vi "CT_DelayPMT_TL_trig.vi"(1 "TL Index":i32=5, 2 "Size of Trig Waveform":dbl=4000.0, 3 "PMT Trig Index":i32=2, 4 "Very Fast Timing In":dbl[](array[slide])=[1100.0, 3200.0, 3254.0, 3290.0, 3100.0, 3080.0, 0.0, 3100.0] min=0.0 max=4000.0 step=2.0 scale=0.0..4000.0 scale format="%#_3f") -> (0 "Very Fast Timing Out":dbl[](array[slide])=[1100.0, 3200.0, 3254.0, 3290.0, 3100.0, 3080.0, 0.0, 3100.0] min=0.0 max=4000.0 step=2.0 scale=0.0..4000.0 scale format="%#_3f")   [LabVIEW 2009]
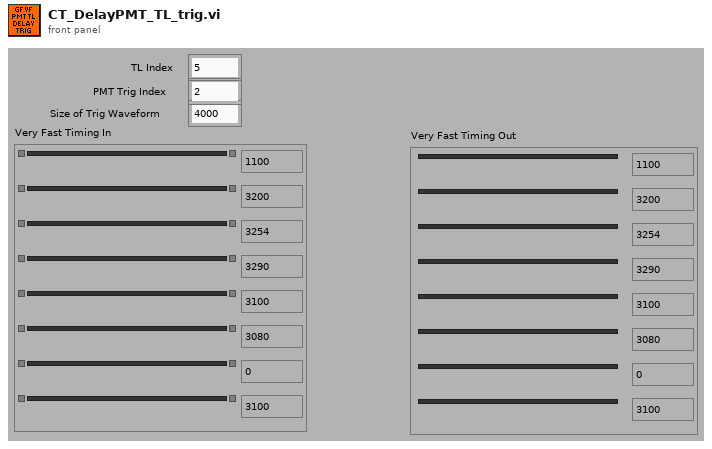
[diagram p1: front panel]
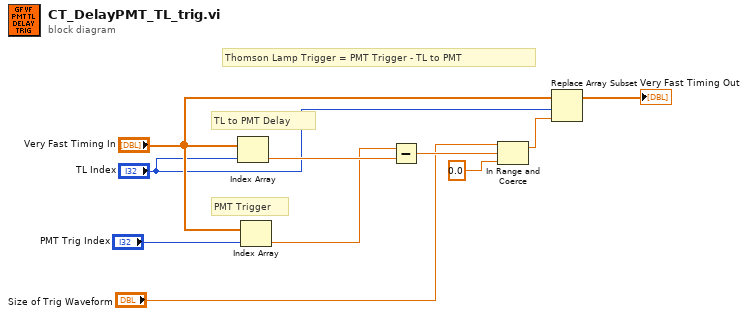
[diagram p0: block diagram]
diagram:
  # "Thomson Lamp Trigger = PMT Trigger - TL to PMT"
  # "PMT Trigger"
  # "TL to PMT Delay"
  n1 = Index Array(array="Very Fast Timing In", index="TL Index") -> (element=w9:dbl)
  n2 = Index Array(array="Very Fast Timing In", index="PMT Trig Index") -> (element=w1:dbl)
  n3 = Subtract(x=w1, y=w9) -> (x-y=w5:dbl)
  n4 = In Range and Coerce(upper limit="Size of Trig Waveform", x=w5, lower limit=0.0) -> (coerced(x)=w4:dbl)  [unwired: 1 out]
  n5 = Replace Array Subset(array="Very Fast Timing In", new element=w4, index="TL Index") -> (→"Very Fast Timing Out":dbl[])
